vi "XML Script - Index 1D Array.vi"(0 "x":i32=-1, 1 "y":i32=-1, 2 "out":i32=-1, 4 "Array Term ID":string, 6 "name":string, 8 "size":i32=1, 9 "prefix (name)":string, 10 "in":i32=-1) -> (5 "Array Element Term IDs":string[](array[string]), 7 "XML Script Command - Index Array":string)   [LabVIEW 2017]
uses:
  <vilib>/_script/XML Scripting/XML Script - Wire (BD).vi
panel:
  # "position"
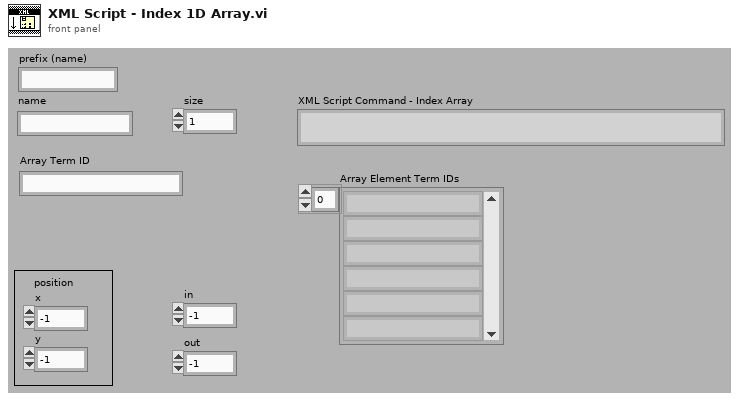
[diagram p1: front panel]
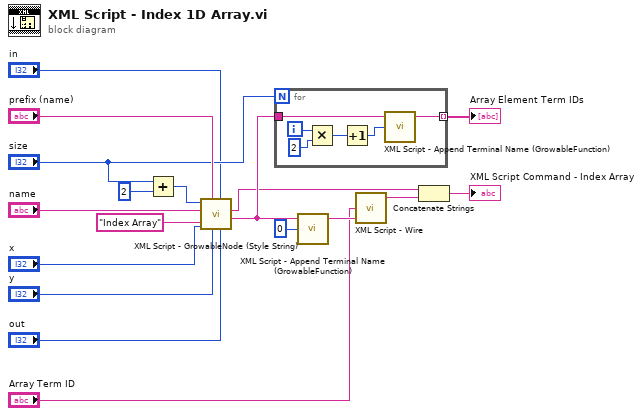
[diagram p0: block diagram]
diagram:
  n1 = Add(x="size", y=2 ("size")) -> (x+y=w17:i32)
  n2 = call <vilib>:"XML Script - GrowableNode (Style String).vi"("x"="x", "y"="y", "out"="out", "Growable Node Style"="Index Array", "name"="name", "size"=w17, "prefix (name)"="prefix (name)", "in"="in") -> ("name (wire source)"=w13:string, "XML Script Command - Growable Node"=w3:string)  [unwired: 2 in]
  n3 = for {
    N: "size" -> [_]
    tunnel: w13 -> [w24]
    tunnel: [w23] -> w7 mode=indexing
    i -> [w22]
    n4 = Multiply(x=w22, y=2 ("size")) -> (x*y=w21:i32)
    n5 = Increment(x=w21) -> (x+1=w20:i32)
    n6 = call <vilib>:"XML Script - Append Terminal Name (GrowableFunction).vi"("i-th term"=w20, "name"=w24) -> ("name.element[i]"=w23:string)  [unwired: 3 out]
  }
  "Array Element Term IDs" <- w7
  n7 = call <vilib>:"XML Script - Append Terminal Name (GrowableFunction).vi"("i-th term"=0, "name"=w13) -> ("name.element[i]"=w6:string)  [unwired: 3 out]
  n8 = call-poly <vilib>:"XML Script - Wire.vi"("destination"=w6, "source"="Array Term ID") -> ("XML Script Command - Wire"=w4:string)  [unwired: 3 out]
  n9 = Concatenate Strings(w3, w4) -> (→"XML Script Command - Index Array":string)
